vi "Goo02.vi"() -> ()   [LabVIEW 2014]
uses:
  <vilib>/myRIO/Instrument Drivers/Onboard IO/AI/vis/Read.vi
  <vilib>/myRIO/Instrument Drivers/Onboard IO/AI/vis/Smart Open.vi
  <vilib>/Utility/error.llb/Error Cluster From Error Code.vi
  <vilib>/myRIO/Common/Instrument Driver Framework/myRIO v1.0/AI/vis/myRIO v1.0 Read AI.vi
panel:
  out "Col02 (B/AI2 (Pin 7)) 2":dbl
  out "숫자형 2":dbl
  out "Col02 (B/AI2 (Pin 7))":dbl
  out "숫자형":dbl
  out "원소의 인덱스":i32
  # "앞의 검은선 수평 맞추기"
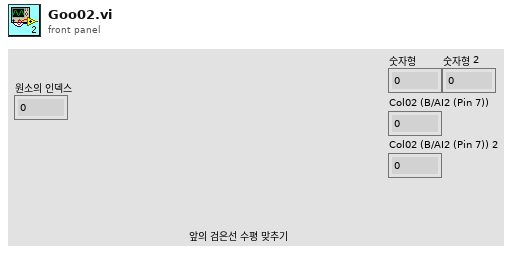
[diagram p1: front panel]
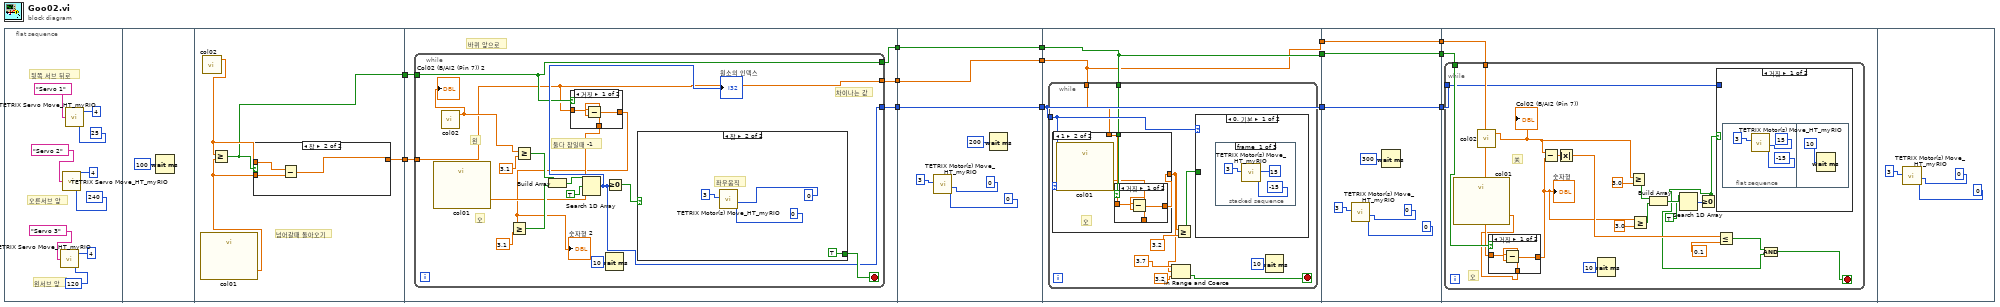
[diagram p0: block diagram]
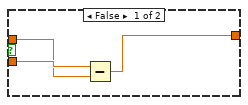
[diagram p2: hidden frame]
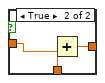
[diagram p3: hidden frame]
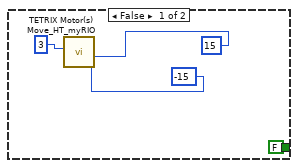
[diagram p4: hidden frame]
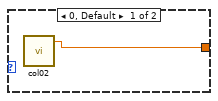
[diagram p5: hidden frame]
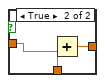
[diagram p6: hidden frame]
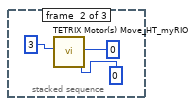
[diagram p7: hidden frame]
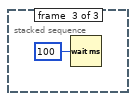
[diagram p8: hidden frame]
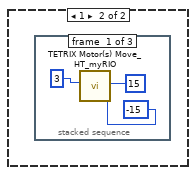
[diagram p9: hidden frame]
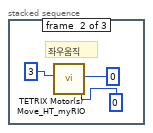
[diagram p10: hidden frame]
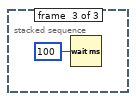
[diagram p11: hidden frame]
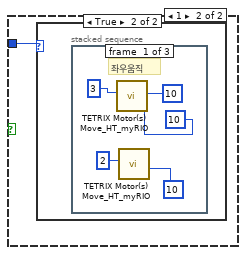
[diagram p12: hidden frame]
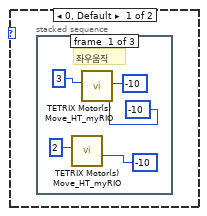
[diagram p13: hidden frame]
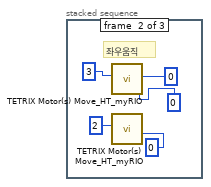
[diagram p14: hidden frame]
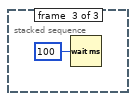
[diagram p15: hidden frame]
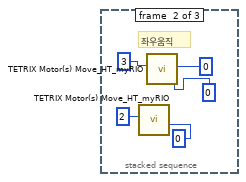
[diagram p16: hidden frame]
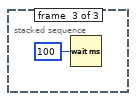
[diagram p17: hidden frame]
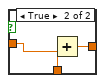
[diagram p18: hidden frame]
diagram:
  n1 = flat-sequence {
    tunnel: [w26] -> w8
    tunnel: [w25] -> w7
    tunnel: [w39] -> w3
    tunnel: [w38] -> w2
    tunnel: [w37] -> w1
    tunnel: w8 -> [w36]
    tunnel: w7 -> [w35]
    tunnel: w3 -> [w75]
    tunnel: [w75] -> w14
    tunnel: w2 -> [w74]
    tunnel: [w74] -> w13
    tunnel: w1 -> [w73]
    tunnel: [w73] -> w12
    tunnel: w14 -> [w78]
    tunnel: [w78] -> w6
    tunnel: w13 -> [w77]
    tunnel: w12 -> [w76]
    tunnel: [w77] -> w5
    tunnel: [w76] -> w4
    tunnel: w6 -> [w120]
    tunnel: [w120] -> w11
    tunnel: w5 -> [w119]
    tunnel: [w119] -> w10
    tunnel: w4 -> [w118]
    tunnel: [w118] -> w9
    tunnel: w11 -> [w123]
    tunnel: w10 -> [w122]
    tunnel: w9 -> [w121]
    frame #0 {
      # "왼서브 앞"
      # "오른서브 앞"
      # "뒷쪽 서브 뒤로"
      n2 = call <vilib>:"TETRIX Servo Move_HT_myRIO.vi"("Servo Position (0 - 255)"=u8 120, "Controller Daisy Chain Position (1 - 4)"=u8 4, "Select Servo"="Servo 3") -> ()  [unwired: 2 in, 1 out]
      n3 = call <vilib>:"TETRIX Servo Move_HT_myRIO.vi"("Servo Position (0 - 255)"=u8 240, "Controller Daisy Chain Position (1 - 4)"=u8 4, "Select Servo"="Servo 2") -> ()  [unwired: 2 in, 1 out]
      n4 = call <vilib>:"TETRIX Servo Move_HT_myRIO.vi"("Servo Position (0 - 255)"=u8 25, "Controller Daisy Chain Position (1 - 4)"=u8 4, "Select Servo"="Servo 1") -> ()  [unwired: 2 in, 1 out]
    }
    frame #1 {
      n5 = Wait (ms)(milliseconds to wait=u32 100 ("대기 시간(ms)")) -> ()  [unwired: 1 out]
    }
    frame #2 {
      # "넘어갈때 돌아오기"
      n6 = call "col01.vi"() -> ("Col01 (B/AI1 (Pin 5))"=w27:dbl)  [unwired: 26 in, 1 out]
      n7 = call "col02.vi"() -> ("Col02 (B/AI2 (Pin 7))"=w28:dbl)  [unwired: 26 in, 1 out]
      n8 = Greater Or Equal?(x=w28, y=w27) -> (x >= y?=w26:bool)
      n9 = case shown="참" w26 {
        tunnel: w28 -> [w30 w34]
        tunnel: w27 -> [w31 w33]
        tunnel: [w29 w32] -> w25
        frame False {
          n10 = Subtract(x=w31, y=w30) -> (x-y=w29:dbl)
        }
        frame True {
          n11 = Subtract(x=w34, y=w33) -> (x-y=w32:dbl)
        }
      }
    }
    frame #3 {
      # "바퀴 앞으로"
      n12 = while {
        tunnel: [w46] -> w39
        tunnel: [w43] -> w38
        tunnel: [w42] -> w37
        tunnel: w36 -> [w43]
        tunnel: w35 -> [w42]
        stop <- w47 stop-if-true
        # "차이나는 값"
        # "오"
        # "왼"
        # "둘다 참일때 -1"
        n13 = call "col01.vi"() -> ("Col01 (B/AI1 (Pin 5))"=w41:dbl)  [unwired: 26 in, 1 out]
        n14 = call "col02.vi"() -> ("Col02 (B/AI2 (Pin 7))"=w44:dbl)  [unwired: 26 in, 1 out]
        "Col02 (B/AI2 (Pin 7)) 2" <- w44
        n15 = Greater Or Equal?(x=w44, y=3.1) -> (x >= y?=w50:bool)
        n16 = case shown="거짓" w43 {
          tunnel: w42 -> [w57 w60]
          tunnel: w41 -> [w56 w59]
          tunnel: [w55 w58] -> w40
          frame False {
            n17 = Subtract(x=w56, y=w57) -> (x-y=w55:dbl)
          }
          frame True {
            n18 = Add(x=w59, y=w60) -> (x+y=w58:dbl)
          }
        }
        "숫자형 2" <- w40
        n19 = Greater Or Equal?(x=w40, y=3.1) -> (x >= y?=w51:bool)
        n20 = Build Array(w50, w51) -> (w54:bool[])
        n21 = Search 1D Array(1D array=w54, element=TRUE ("원소")) -> (index of element=w46:i32)  [unwired: 1 in]
        "원소의 인덱스" <- w46
        n22 = Wait (ms)(milliseconds to wait=u32 10 ("대기 시간(ms)")) -> ()  [unwired: 1 out]
        n23 = Greater Or Equal To 0?(x=w46) -> (x >= 0?=w52:bool)
        n24 = case shown="참" w52 {
          tunnel: [FALSE TRUE] -> w47
          frame False {
            n25 = call <vilib>:"TETRIX Motor(s) Move_HT_myRIO.vi"("Motor 2 Power (-100 to 100)\n0 = Stop/Brake\n-128 = Stop/Coast"=i8 -15 ("Motor 2 Power (-100 to 100)\n0 = Stop/Brake\n-128 = Stop/Coast"), "Motor 1 Power (-100 to 100)\n0 = Stop/Brake\n-128 = Stop/Coast"=i8 15 ("Motor 1 Power (-100 to 100)\n0 = Stop/Brake\n-128 = Stop/Coast"), "Controller Daisy Chain Position: 1 - 4"=u8 3) -> ()  [unwired: 6 in, 1 out]
          }
          frame True {
            # "좌우움직"
            n26 = call <vilib>:"TETRIX Motor(s) Move_HT_myRIO.vi"("Motor 2 Power (-100 to 100)\n0 = Stop/Brake\n-128 = Stop/Coast"=i8 0 ("Motor 2 Power (-100 to 100)\n0 = Stop/Brake\n-128 = Stop/Coast"), "Motor 1 Power (-100 to 100)\n0 = Stop/Brake\n-128 = Stop/Coast"=i8 0 ("Motor 1 Power (-100 to 100)\n0 = Stop/Brake\n-128 = Stop/Coast"), "Controller Daisy Chain Position: 1 - 4"=u8 3) -> ()  [unwired: 6 in, 1 out]
          }
        }
      }
    }
    frame #4 {
      n27 = call <vilib>:"TETRIX Motor(s) Move_HT_myRIO.vi"("Motor 2 Power (-100 to 100)\n0 = Stop/Brake\n-128 = Stop/Coast"=i8 0 ("Motor 2 Power (-100 to 100)\n0 = Stop/Brake\n-128 = Stop/Coast"), "Motor 1 Power (-100 to 100)\n0 = Stop/Brake\n-128 = Stop/Coast"=i8 0 ("Motor 1 Power (-100 to 100)\n0 = Stop/Brake\n-128 = Stop/Coast"), "Controller Daisy Chain Position: 1 - 4"=u8 3) -> ()  [unwired: 6 in, 1 out]
      n28 = Wait (ms)(milliseconds to wait=u32 200 ("대기 시간(ms)")) -> ()  [unwired: 1 out]
    }
    frame #5 {
      n29 = while {
        tunnel: w78 -> [w88]
        tunnel: w76 -> [w80]
        tunnel: w77 -> [w81]
        stop <- w87 stop-if-true
        n30 = case shown="1" w88 {
          tunnel: [w89 w93] -> w82
          tunnel: w81 -> [_ w92]
          tunnel: w80 -> [_ w91]
          frame 0, Default {
            n31 = call "col02.vi"() -> ("Col02 (B/AI2 (Pin 7))"=w89:dbl)  [unwired: 26 in, 1 out]
          }
          frame 1 {
            # "오"
            n32 = call "col01.vi"() -> ("Col01 (B/AI1 (Pin 5))"=w90:dbl)  [unwired: 26 in, 1 out]
            n33 = case shown="거짓" w92 {
              tunnel: w91 -> [w96 w99]
              tunnel: w90 -> [w95 w98]
              tunnel: [w94 w97] -> w93
              frame False {
                n34 = Subtract(x=w95, y=w96) -> (x-y=w94:dbl)
              }
              frame True {
                n35 = Add(x=w98, y=w99) -> (x+y=w97:dbl)
              }
            }
          }
        }
        n36 = In Range and Coerce(upper limit=3.7 ("y"), x=w82, lower limit=3.2 ("하위 리미트")) -> (In Range?=w87:bool)  [unwired: 1 out]
        n37 = Greater Or Equal?(x=w82, y=3.2) -> (x >= y?=w83:bool)
        n38 = case shown="0, 기본" w88 {
          tunnel: w83 -> [_ _]
          frame 0, Default {
            n39 = stacked-sequence {
              frame #0 {
                n40 = call <vilib>:"TETRIX Motor(s) Move_HT_myRIO.vi"("Motor 2 Power (-100 to 100)\n0 = Stop/Brake\n-128 = Stop/Coast"=i8 -15 ("Motor 2 Power (-100 to 100)\n0 = Stop/Brake\n-128 = Stop/Coast"), "Motor 1 Power (-100 to 100)\n0 = Stop/Brake\n-128 = Stop/Coast"=i8 15 ("Motor 1 Power (-100 to 100)\n0 = Stop/Brake\n-128 = Stop/Coast"), "Controller Daisy Chain Position: 1 - 4"=u8 3) -> ()  [unwired: 6 in, 1 out]
              }
              frame #1 {
                n41 = call <vilib>:"TETRIX Motor(s) Move_HT_myRIO.vi"("Motor 2 Power (-100 to 100)\n0 = Stop/Brake\n-128 = Stop/Coast"=i8 0 ("Motor 2 Power (-100 to 100)\n0 = Stop/Brake\n-128 = Stop/Coast"), "Motor 1 Power (-100 to 100)\n0 = Stop/Brake\n-128 = Stop/Coast"=i8 0 ("Motor 1 Power (-100 to 100)\n0 = Stop/Brake\n-128 = Stop/Coast"), "Controller Daisy Chain Position: 1 - 4"=u8 3) -> ()  [unwired: 6 in, 1 out]
              }
              frame #2 {
                n42 = Wait (ms)(milliseconds to wait=u32 100 ("대기 시간(ms)")) -> ()  [unwired: 1 out]
              }
            }
          }
          frame 1 {
            n43 = stacked-sequence {
              frame #0 {
                n44 = call <vilib>:"TETRIX Motor(s) Move_HT_myRIO.vi"("Motor 2 Power (-100 to 100)\n0 = Stop/Brake\n-128 = Stop/Coast"=i8 -15 ("Motor 2 Power (-100 to 100)\n0 = Stop/Brake\n-128 = Stop/Coast"), "Motor 1 Power (-100 to 100)\n0 = Stop/Brake\n-128 = Stop/Coast"=i8 15 ("Motor 1 Power (-100 to 100)\n0 = Stop/Brake\n-128 = Stop/Coast"), "Controller Daisy Chain Position: 1 - 4"=u8 3) -> ()  [unwired: 6 in, 1 out]
              }
              frame #1 {
                # "좌우움직"
                n45 = call <vilib>:"TETRIX Motor(s) Move_HT_myRIO.vi"("Motor 2 Power (-100 to 100)\n0 = Stop/Brake\n-128 = Stop/Coast"=i8 0 ("Motor 2 Power (-100 to 100)\n0 = Stop/Brake\n-128 = Stop/Coast"), "Motor 1 Power (-100 to 100)\n0 = Stop/Brake\n-128 = Stop/Coast"=i8 0 ("Motor 1 Power (-100 to 100)\n0 = Stop/Brake\n-128 = Stop/Coast"), "Controller Daisy Chain Position: 1 - 4"=u8 3) -> ()  [unwired: 6 in, 1 out]
              }
              frame #2 {
                n46 = Wait (ms)(milliseconds to wait=u32 100 ("대기 시간(ms)")) -> ()  [unwired: 1 out]
              }
            }
          }
        }
        n47 = Wait (ms)(milliseconds to wait=u32 10 ("대기 시간(ms)")) -> ()  [unwired: 1 out]
      }
    }
    frame #6 {
      n48 = call <vilib>:"TETRIX Motor(s) Move_HT_myRIO.vi"("Motor 2 Power (-100 to 100)\n0 = Stop/Brake\n-128 = Stop/Coast"=i8 0 ("Motor 2 Power (-100 to 100)\n0 = Stop/Brake\n-128 = Stop/Coast"), "Motor 1 Power (-100 to 100)\n0 = Stop/Brake\n-128 = Stop/Coast"=i8 0 ("Motor 1 Power (-100 to 100)\n0 = Stop/Brake\n-128 = Stop/Coast"), "Controller Daisy Chain Position: 1 - 4"=u8 3) -> ()  [unwired: 6 in, 1 out]
      n49 = Wait (ms)(milliseconds to wait=u32 300 ("대기 시간(ms)")) -> ()  [unwired: 1 out]
    }
    frame #7 {
      n50 = while {
        tunnel: w123 -> [w124]
        tunnel: w122 -> [w140]
        tunnel: w121 -> [w139]
        stop <- w126 stop-if-true
        # "오"
        # "关"
        n51 = call "col01.vi"() -> ("Col01 (B/AI1 (Pin 5))"=w138:dbl)  [unwired: 26 in, 1 out]
        n52 = call "col02.vi"() -> ("Col02 (B/AI2 (Pin 7))"=w134:dbl)  [unwired: 26 in, 1 out]
        "Col02 (B/AI2 (Pin 7))" <- w134
        n53 = case shown="거짓" w140 {
          tunnel: w139 -> [w173 w176]
          tunnel: w138 -> [w172 w175]
          tunnel: [w171 w174] -> w133
          frame False {
            n54 = Subtract(x=w172, y=w173) -> (x-y=w171:dbl)
          }
          frame True {
            n55 = Add(x=w175, y=w176) -> (x+y=w174:dbl)
          }
        }
        "숫자형" <- w133
        n56 = Subtract(x=w134, y=w133) -> (x-y=w143:dbl)
        n57 = Absolute Value(x=w143) -> (abs(x)=w142:dbl)
        n58 = Wait (ms)(milliseconds to wait=u32 10 ("대기 시간(ms)")) -> ()  [unwired: 1 out]
        n59 = Greater Or Equal?(x=w134, y=3.0) -> (x >= y?=w132:bool)
        n60 = Greater Or Equal?(x=w133, y=3.0) -> (x >= y?=w131:bool)
        n61 = Build Array(w132, w131) -> (w130:bool[])
        n62 = Search 1D Array(1D array=w130, element=TRUE ("원소")) -> (index of element=w125:i32)  [unwired: 1 in]
        n63 = Greater Or Equal To 0?(x=w125) -> (x >= 0?=w127:bool)
        n64 = case shown="거짓" w127 {
          tunnel: w124 -> [_ w148]
          frame False {
            n65 = flat-sequence {
              frame #0 {
                n66 = call <vilib>:"TETRIX Motor(s) Move_HT_myRIO.vi"("Motor 2 Power (-100 to 100)\n0 = Stop/Brake\n-128 = Stop/Coast"=i8 -15 ("Motor 2 Power (-100 to 100)\n0 = Stop/Brake\n-128 = Stop/Coast"), "Motor 1 Power (-100 to 100)\n0 = Stop/Brake\n-128 = Stop/Coast"=i8 15 ("Motor 1 Power (-100 to 100)\n0 = Stop/Brake\n-128 = Stop/Coast"), "Controller Daisy Chain Position: 1 - 4"=u8 3) -> ()  [unwired: 6 in, 1 out]
              }
              frame #1 {
                n67 = Wait (ms)(milliseconds to wait=u32 10 ("ms 타이머 값")) -> ()  [unwired: 1 out]
              }
            }
          }
          frame True {
            n68 = case shown="1" w148 {
              frame 0, Default {
                n69 = stacked-sequence {
                  frame #0 {
                    # "좌우움직"
                    n70 = call <vilib>:"TETRIX Motor(s) Move_HT_myRIO.vi"("Motor 1 Power (-100 to 100)\n0 = Stop/Brake\n-128 = Stop/Coast"=i8 -10 ("Motor 1 Power (-100 to 100)\n0 = Stop/Brake\n-128 = Stop/Coast"), "Controller Daisy Chain Position: 1 - 4"=u8 2) -> ()  [unwired: 7 in, 1 out]
                    n71 = call <vilib>:"TETRIX Motor(s) Move_HT_myRIO.vi"("Motor 2 Power (-100 to 100)\n0 = Stop/Brake\n-128 = Stop/Coast"=i8 -10 ("Motor 2 Power (-100 to 100)\n0 = Stop/Brake\n-128 = Stop/Coast"), "Motor 1 Power (-100 to 100)\n0 = Stop/Brake\n-128 = Stop/Coast"=i8 -10 ("Motor 1 Power (-100 to 100)\n0 = Stop/Brake\n-128 = Stop/Coast"), "Controller Daisy Chain Position: 1 - 4"=u8 3) -> ()  [unwired: 6 in, 1 out]
                  }
                  frame #1 {
                    # "좌우움직"
                    n72 = call <vilib>:"TETRIX Motor(s) Move_HT_myRIO.vi"("Motor 2 Power (-100 to 100)\n0 = Stop/Brake\n-128 = Stop/Coast"=i8 0 ("Motor 2 Power (-100 to 100)\n0 = Stop/Brake\n-128 = Stop/Coast"), "Motor 1 Power (-100 to 100)\n0 = Stop/Brake\n-128 = Stop/Coast"=i8 0 ("Motor 1 Power (-100 to 100)\n0 = Stop/Brake\n-128 = Stop/Coast"), "Controller Daisy Chain Position: 1 - 4"=u8 3) -> ()  [unwired: 6 in, 1 out]
                    n73 = call <vilib>:"TETRIX Motor(s) Move_HT_myRIO.vi"("Motor 1 Power (-100 to 100)\n0 = Stop/Brake\n-128 = Stop/Coast"=i8 0 ("Motor 1 Power (-100 to 100)\n0 = Stop/Brake\n-128 = Stop/Coast"), "Controller Daisy Chain Position: 1 - 4"=u8 2) -> ()  [unwired: 7 in, 1 out]
                  }
                  frame #2 {
                    n74 = Wait (ms)(milliseconds to wait=u32 100 ("대기 시간(ms)")) -> ()  [unwired: 1 out]
                  }
                }
              }
              frame 1 {
                n75 = stacked-sequence {
                  frame #0 {
                    # "좌우움직"
                    n76 = call <vilib>:"TETRIX Motor(s) Move_HT_myRIO.vi"("Motor 2 Power (-100 to 100)\n0 = Stop/Brake\n-128 = Stop/Coast"=i8 10 ("Motor 2 Power (-100 to 100)\n0 = Stop/Brake\n-128 = Stop/Coast"), "Motor 1 Power (-100 to 100)\n0 = Stop/Brake\n-128 = Stop/Coast"=i8 10 ("Motor 1 Power (-100 to 100)\n0 = Stop/Brake\n-128 = Stop/Coast"), "Controller Daisy Chain Position: 1 - 4"=u8 3) -> ()  [unwired: 6 in, 1 out]
                    n77 = call <vilib>:"TETRIX Motor(s) Move_HT_myRIO.vi"("Motor 1 Power (-100 to 100)\n0 = Stop/Brake\n-128 = Stop/Coast"=i8 10 ("Motor 1 Power (-100 to 100)\n0 = Stop/Brake\n-128 = Stop/Coast"), "Controller Daisy Chain Position: 1 - 4"=u8 2) -> ()  [unwired: 7 in, 1 out]
                  }
                  frame #1 {
                    # "좌우움직"
                    n78 = call <vilib>:"TETRIX Motor(s) Move_HT_myRIO.vi"("Motor 1 Power (-100 to 100)\n0 = Stop/Brake\n-128 = Stop/Coast"=i8 0 ("Motor 1 Power (-100 to 100)\n0 = Stop/Brake\n-128 = Stop/Coast"), "Controller Daisy Chain Position: 1 - 4"=u8 2) -> ()  [unwired: 7 in, 1 out]
                    n79 = call <vilib>:"TETRIX Motor(s) Move_HT_myRIO.vi"("Motor 2 Power (-100 to 100)\n0 = Stop/Brake\n-128 = Stop/Coast"=i8 0 ("Motor 2 Power (-100 to 100)\n0 = Stop/Brake\n-128 = Stop/Coast"), "Motor 1 Power (-100 to 100)\n0 = Stop/Brake\n-128 = Stop/Coast"=i8 0 ("Motor 1 Power (-100 to 100)\n0 = Stop/Brake\n-128 = Stop/Coast"), "Controller Daisy Chain Position: 1 - 4"=u8 3) -> ()  [unwired: 6 in, 1 out]
                  }
                  frame #2 {
                    n80 = Wait (ms)(milliseconds to wait=u32 100 ("대기 시간(ms)")) -> ()  [unwired: 1 out]
                  }
                }
              }
            }
          }
        }
        n81 = Less Or Equal?(x=w142, y=0.1) -> (x <= y?=w128:bool)
        n82 = And(x=w128, y=w127) -> (x .and. y?=w126:bool)
      }
    }
    frame #8 {
      n83 = call <vilib>:"TETRIX Motor(s) Move_HT_myRIO.vi"("Motor 2 Power (-100 to 100)\n0 = Stop/Brake\n-128 = Stop/Coast"=i8 0 ("Motor 2 Power (-100 to 100)\n0 = Stop/Brake\n-128 = Stop/Coast"), "Motor 1 Power (-100 to 100)\n0 = Stop/Brake\n-128 = Stop/Coast"=i8 0 ("Motor 1 Power (-100 to 100)\n0 = Stop/Brake\n-128 = Stop/Coast"), "Controller Daisy Chain Position: 1 - 4"=u8 3) -> ()  [unwired: 6 in, 1 out]
    }
  }
